vi "7.vi"() -> ()   [LabVIEW 2020]
panel:
  in  "Numeric":dbl
  out "s? t:f":string
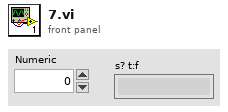
[diagram p1: front panel]
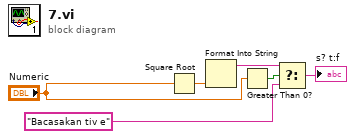
[diagram p0: block diagram]
diagram:
  n1 = Square Root(x="Numeric") -> (sqrt(x)=w6:dbl)
  n2 = Format Into String(w6) -> (resulting string=w5:string)  [unwired: 3 in, 1 out]
  n3 = Greater Than 0?(x="Numeric") -> (x > 0?=w2:bool)
  n4 = Select(t=w5, s=w2, f="Bacasakan tiv e") -> (s? t:f=→"s? t:f":string)
